vi "Set Vehicle Speed Override.vi"(6 "error in":errorcluster, 7 "DATA[5]":u8=3 format="%.0x", 8 "MaxRead":i32, 9 "Channel in":u16) -> (0 "error out":errorcluster, 1 "Messages":T1(array[cluster]), 2 "Pass":bool, 3 "Channel out":u16)   [LabVIEW 2023]
uses:
  be2a90bf-c340-472d-9dbd-2edbd756b5ea.vi
  3dbf7838-bdc4-4026-8e26-6a8edd8751fd.vi
  51672023-2b8f-422d-bba0-9ae07ec01481.vi
  7f12b63b-630a-4c96-8822-8a95c7c2d06d.vi
  Communication/PCAN2023/PCAN API.lvlib
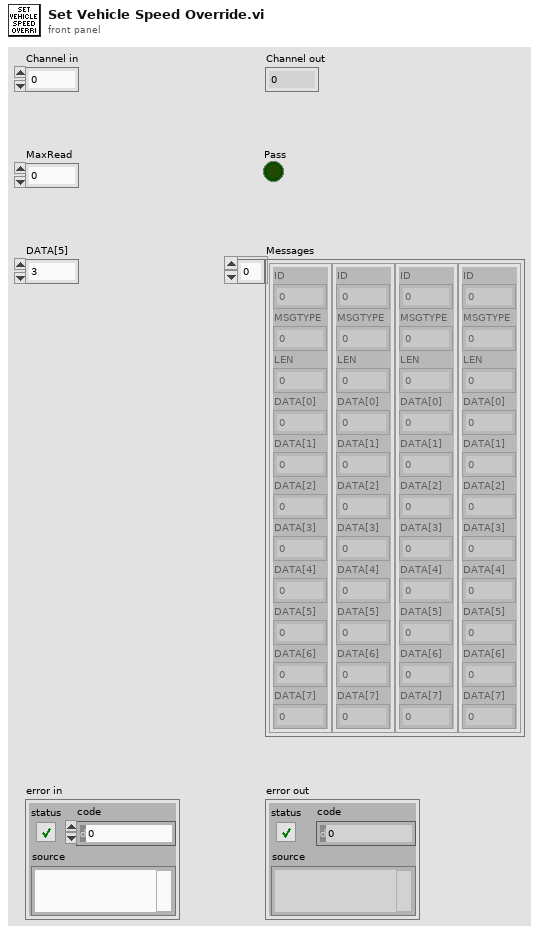
[diagram p1: front panel]
types:
  T1 = cluster{"ID":u32, "MSGTYPE":u8, "LEN":u8, "DATA[0]":u8, "DATA[1]":u8, "DATA[2]":u8, "DATA[3]":u8, "DATA[4]":u8, "DATA[5]":u8, "DATA[6]":u8, "DATA[7]":u8}[]
  T2 = cluster{"ID":u32, "MSGTYPE":u8, "LEN":u8, "DATA[0]":u8, "DATA[1]":u8, "DATA[2]":u8, "DATA[3]":u8, "DATA[4]":u8, "DATA[5]":u8, "DATA[6]":u8, "DATA[7]":u8}
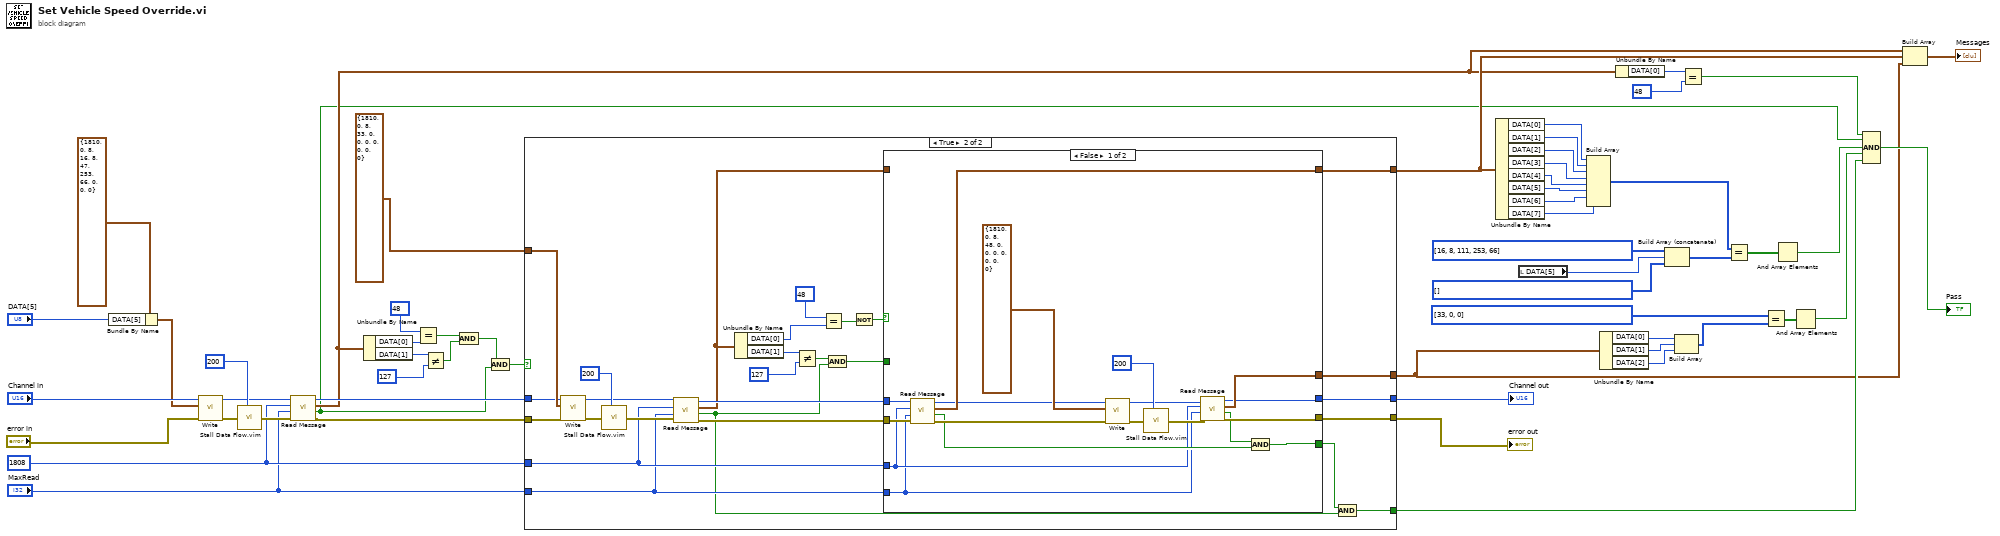
[diagram p0: block diagram]
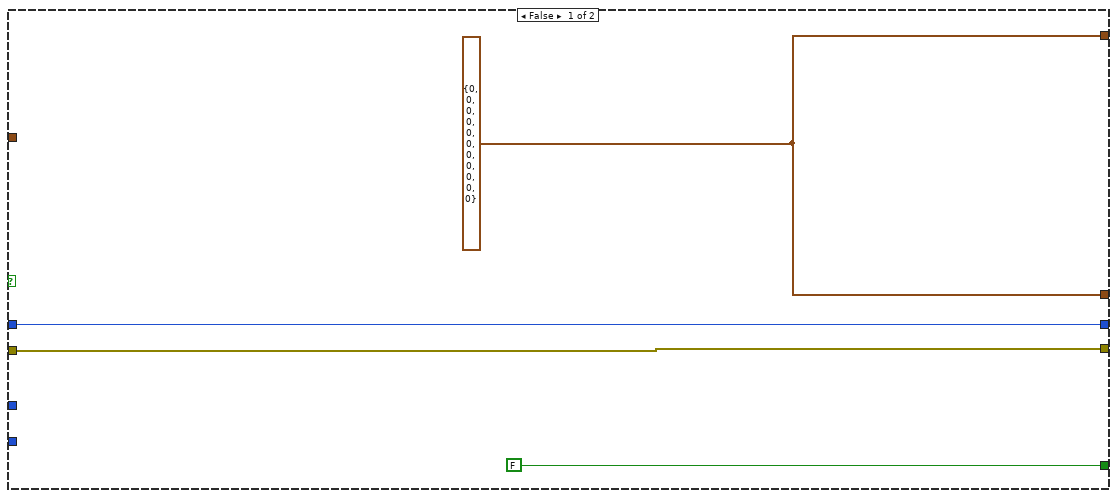
[diagram p2: hidden frame]
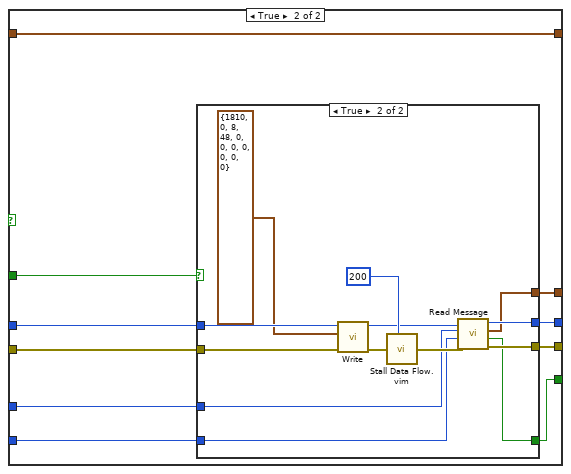
[diagram p3: hidden frame]
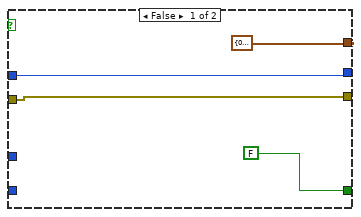
[diagram p4: hidden frame]
diagram:
  w13 = u32 1808 ("ID")
  n1 = Bundle By Name(cluster=T2 {"ID"=1810, "MSGTYPE"=0, "LEN"=8, "DATA[0]"=16, "DATA[1]"=8, "DATA[2]"=47, "DATA[3]"=253, "DATA[4]"=66, "DATA[5]"=0, "DATA[6]"=0, "DATA[7]"=0} ("MessageBuffer"), "DATA[5]"="DATA[5]") -> (w23:T2)
  n2 = call "Write.vi"("error in"="error in", "MessageBuffer"=w23, "Channel"="Channel in") -> ("error out"=w55:errorcluster, "Channel out"=w17:u16)  [unwired: 5 in, 2 out]
  n3 = call "Stall Data Flow.vim"("value in"=w55, "milliseconds to wait"=u32 200) -> ("value out"=w15:errorcluster)  [unwired: 1 out]
  n4 = call "Read Message.vi"("error in"=w15, "MaxRead"="MaxRead", "ID"=w13, "Channel in"=w17) -> ("error out"=w14:errorcluster, "Passed"=w2:bool, "Last Message"=w12:T2, "Channel out"=w16:u16)  [unwired: 3 in, 1 out]
  n5 = Unbundle By Name(w12) -> ("DATA[0]"=w7:u8, "DATA[1]"=w19:u8)
  n6 = Equal?(x=u8 48, y=w7) -> (x = y?=w5:bool)
  n7 = Not Equal?(x=w19, y=u8 127) -> (x != y?=w4:bool)
  n8 = And(x=w5, y=w4) -> (x .and. y?=w3:bool)
  n9 = And(x=w3, y=w2) -> (x .and. y?=w1:bool)
  n10 = case shown="True" w1 {
    tunnel: T2 {"ID"=1810, "MSGTYPE"=0, "LEN"=8, "DATA[0]"=33, "DATA[1]"=0, "DATA[2]"=0, "DATA[3]"=0, "DATA[4]"=0, "DATA[5]"=0, "DATA[6]"=0, "DATA[7]"=0} ("MessageBuffer") -> [_ w86]
    tunnel: w16 -> [w59 w84]
    tunnel: w14 -> [w58 w83]
    tunnel: [w58 w82] -> w45
    tunnel: w13 -> [_ w73]
    tunnel: [w59 w81] -> w44
    tunnel: [FALSE w70] -> w29
    tunnel: [w60 w61] -> w28
    tunnel: [w60 w80] -> w27
    tunnel: "MaxRead" -> [_ w72]
    frame False {
      w60 = T2 {"ID"=0, "MSGTYPE"=0, "LEN"=0, "DATA[0]"=0, "DATA[1]"=0, "DATA[2]"=0, "DATA[3]"=0, "DATA[4]"=0, "DATA[5]"=0, "DATA[6]"=0, "DATA[7]"=0} ("MessageBuffer out")
    }
    frame True {
      n11 = call "Write.vi"("error in"=w83, "MessageBuffer"=w86, "Channel"=w84) -> ("error out"=w85:errorcluster, "Channel out"=w77:u16)  [unwired: 5 in, 2 out]
      n12 = call "Stall Data Flow.vim"("value in"=w85, "milliseconds to wait"=u32 200) -> ("value out"=w76:errorcluster)  [unwired: 1 out]
      n13 = call "Read Message.vi"("error in"=w76, "MaxRead"=w72, "ID"=w73, "Channel in"=w77) -> ("error out"=w74:errorcluster, "Passed"=w68:bool, "Last Message"=w62:T2, "Channel out"=w75:u16)  [unwired: 3 in, 1 out]
      n14 = Unbundle By Name(w62) -> ("DATA[0]"=w65:u8, "DATA[1]"=w78:u8)
      n15 = Not Equal?(x=w78, y=u8 127) -> (x != y?=w69:bool)
      n16 = Equal?(x=u8 48, y=w65) -> (x = y?=w64:bool)
      n17 = And(x=w69, y=w68) -> (x .and. y?=w67:bool)
      n18 = Not(x=w64) -> (.not. x?=w63:bool)
      n19 = case shown="False" w63 {
        tunnel: [w93 w115] -> w82
        tunnel: [w94 w114] -> w81
        tunnel: [w95 w113] -> w80
        tunnel: w75 -> [w104 w112]
        tunnel: w74 -> [w105 w111]
        tunnel: w73 -> [w89 w110]
        tunnel: w72 -> [w88 w109]
        tunnel: [w90 w108] -> w71
        tunnel: w67 -> [_ w107]
        tunnel: w62 -> [_ w106]
        tunnel: [w103 w106] -> w61
        frame False {
          n20 = call "Read Message.vi"("error in"=w105, "MaxRead"=w88, "ID"=w89, "Channel in"=w104) -> ("error out"=w96:errorcluster, "Passed"=w91:bool, "Last Message"=w103:T2, "Channel out"=w97:u16)  [unwired: 3 in, 1 out]
          n21 = call "Write.vi"("error in"=w96, "MessageBuffer"=T2 {"ID"=1810, "MSGTYPE"=0, "LEN"=8, "DATA[0]"=48, "DATA[1]"=0, "DATA[2]"=0, "DATA[3]"=0, "DATA[4]"=0, "DATA[5]"=0, "DATA[6]"=0, "DATA[7]"=0}, "Channel"=w97) -> ("error out"=w102:errorcluster, "Channel out"=w100:u16)  [unwired: 5 in, 2 out]
          n22 = call "Stall Data Flow.vim"("value in"=w102, "milliseconds to wait"=u32 200) -> ("value out"=w99:errorcluster)  [unwired: 1 out]
          n23 = call "Read Message.vi"("error in"=w99, "MaxRead"=w88, "ID"=w89, "Channel in"=w100) -> ("error out"=w93:errorcluster, "Passed"=w92:bool, "Last Message"=w95:T2, "Channel out"=w94:u16)  [unwired: 3 in, 1 out]
          n24 = And(x=w92, y=w91) -> (x .and. y?=w90:bool)
        }
        frame True {
          n25 = case shown="True" w107 {
            tunnel: w112 -> [w119 w130]
            tunnel: w111 -> [w117 w129]
            tunnel: [w117 w125] -> w115
            tunnel: [w119 w126] -> w114
            tunnel: [FALSE w123] -> w108
            tunnel: [T2 {"ID"=0, "MSGTYPE"=0, "LEN"=0, "DATA[0]"=0, "DATA[1]"=0, "DATA[2]"=0, "DATA[3]"=0, "DATA[4]"=0, "DATA[5]"=0, "DATA[6]"=0, "DATA[7]"=0} ("MessageBuffer out") w124] -> w113
            tunnel: w110 -> [_ w122]
            tunnel: w109 -> [_ w121]
            frame False {
            }
            frame True {
              n26 = call "Write.vi"("error in"=w129, "MessageBuffer"=T2 {"ID"=1810, "MSGTYPE"=0, "LEN"=8, "DATA[0]"=48, "DATA[1]"=0, "DATA[2]"=0, "DATA[3]"=0, "DATA[4]"=0, "DATA[5]"=0, "DATA[6]"=0, "DATA[7]"=0}, "Channel"=w130) -> ("error out"=w132:errorcluster, "Channel out"=w128:u16)  [unwired: 5 in, 2 out]
              n27 = call "Stall Data Flow.vim"("value in"=w132, "milliseconds to wait"=u32 200) -> ("value out"=w127:errorcluster)  [unwired: 1 out]
              n28 = call "Read Message.vi"("error in"=w127, "MaxRead"=w121, "ID"=w122, "Channel in"=w128) -> ("error out"=w125:errorcluster, "Passed"=w123:bool, "Last Message"=w124:T2, "Channel out"=w126:u16)  [unwired: 3 in, 1 out]
            }
          }
        }
      }
      n29 = And(x=w71, y=w68) -> (x .and. y?=w70:bool)
    }
  }
  "error out" <- w45
  "Channel out" <- w44
  n30 = Unbundle By Name(w28) -> ("DATA[0]"=w41:u8, "DATA[1]"=w50:u8, "DATA[2]"=w49:u8, "DATA[3]"=w48:u8, "DATA[4]"=w47:u8, "DATA[5]"=w40:u8, "DATA[6]"=w39:u8, "DATA[7]"=w38:u8)
  n31 = local read "DATA[5]"() -> (w21:u8)
  n32 = Build Array(w41, w50, w49, w48, w47, w40, w39, w38) -> (w9:u8[])
  n33 = Unbundle By Name(w27) -> ("DATA[0]"=w37:u8, "DATA[1]"=w36:u8, "DATA[2]"=w35:u8)
  n34 = Unbundle By Name(w12) -> ("DATA[0]"=w43:u8)
  n35 = Build Array (concatenate)(u8[] [16, 8, 111, 253, 66] ("x"), w21, u8[] [] ("x")) -> (w10:u8[])
  n36 = Build Array(w37, w36, w35) -> (w33:u8[])
  n37 = Equal?(x=w43, y=u8 48) -> (x = y?=w31:bool)
  n38 = Equal?(x=w9, y=w10) -> (x = y?=w53:bool[])
  n39 = Equal?(x=u8[] [33, 0, 0], y=w33) -> (x = y?=w32:bool[])
  n40 = And Array Elements(Boolean array=w53) -> (logical AND=w8:bool)
  n41 = And Array Elements(Boolean array=w32) -> (logical AND=w30:bool)
  n42 = Compound Arithmetic op=AND(w31, w2, w8, w30, w29) -> (→"Pass":bool)
  n43 = Build Array(w12, w28, w27) -> (→"Messages":T1)
